vi "LWXPS_PositionerPositionCompareEnable.vi"(6 "LabVIEW error IN":errorcluster, 8 "Positioner Name":string, 9 "XPS Reference IN":refnum<k24>) -> (0 "LabVIEW error OUT":errorcluster, 1 "XPS Error String":string, 2 "Returned error code":i32, 3 "XPS Reference OUT":refnum<k24>)   [LabVIEW 2015]
uses:
  D:/labview program/whole brain TP_221122_xz/sub vi/XPS-UNIFIED/LabVIEW VIs/LabVIEW Source Code/Dll/Newport.XPS.CommandInterface.dll
  Dll/Newport.XPS.CommandInterface.dll
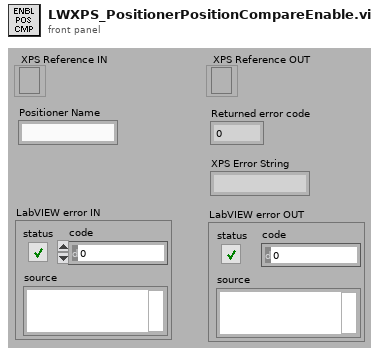
[diagram p1: front panel]
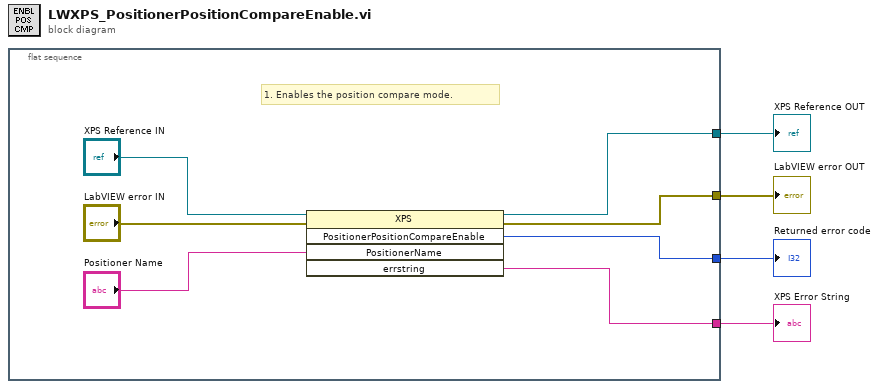
[diagram p0: block diagram]
diagram:
  n1 = flat-sequence {
    tunnel: [w5] -> w1
    tunnel: [w10] -> w4
    tunnel: [w9] -> w3
    tunnel: [w8] -> w2
    frame #0 {
      # "1. Enables the position compare mode."
      n2 = invoke class="XPS" method="PositionerPositionCompareEnable"(reference="XPS Reference IN", error in="LabVIEW error IN", "PositionerName"="Positioner Name") -> (reference out=w10:refnum<k24>, error out=w9:errorcluster, "PositionerPositionCompareEnable"=w8:i32, "errstring"=w5:string)  [unwired: 2 in, 1 out]
    }
  }
  "XPS Error String" <- w1
  "XPS Reference OUT" <- w4
  "LabVIEW error OUT" <- w3
  "Returned error code" <- w2
